vi "file -- accumulate data files -- V5.vi"(11 "list of <mmddyy> folders":path[](array[path])) -> (0 "timestamp (min) array":dbl[](array[numeric]), 2 "sweep file name  array":T1[](array[typedef]))   [LabVIEW 2015]
uses:
  sweep file name.ctl
  file -- scan filename action.ctl
  Split file name.vi
  find all matching strings in the list.vi
panel:
  in  "dummy":T1={"temperature"=0.0, "temperature str"="", "file path"=path "/snowfall/Users/arcadi/Desktop/Ultrasound/Experiment/YBCO_4/Round1/Sweep12/June_2011/062511/221.16400K_300_3100_001_062511.dat", "last mod"=timestamp(0 s since 1904-01-01), "file name str"="", "mod time(min)"=0.0, "file format"=enum."", "power(V)"=0.0, "Magn Field(T) "=0.0}
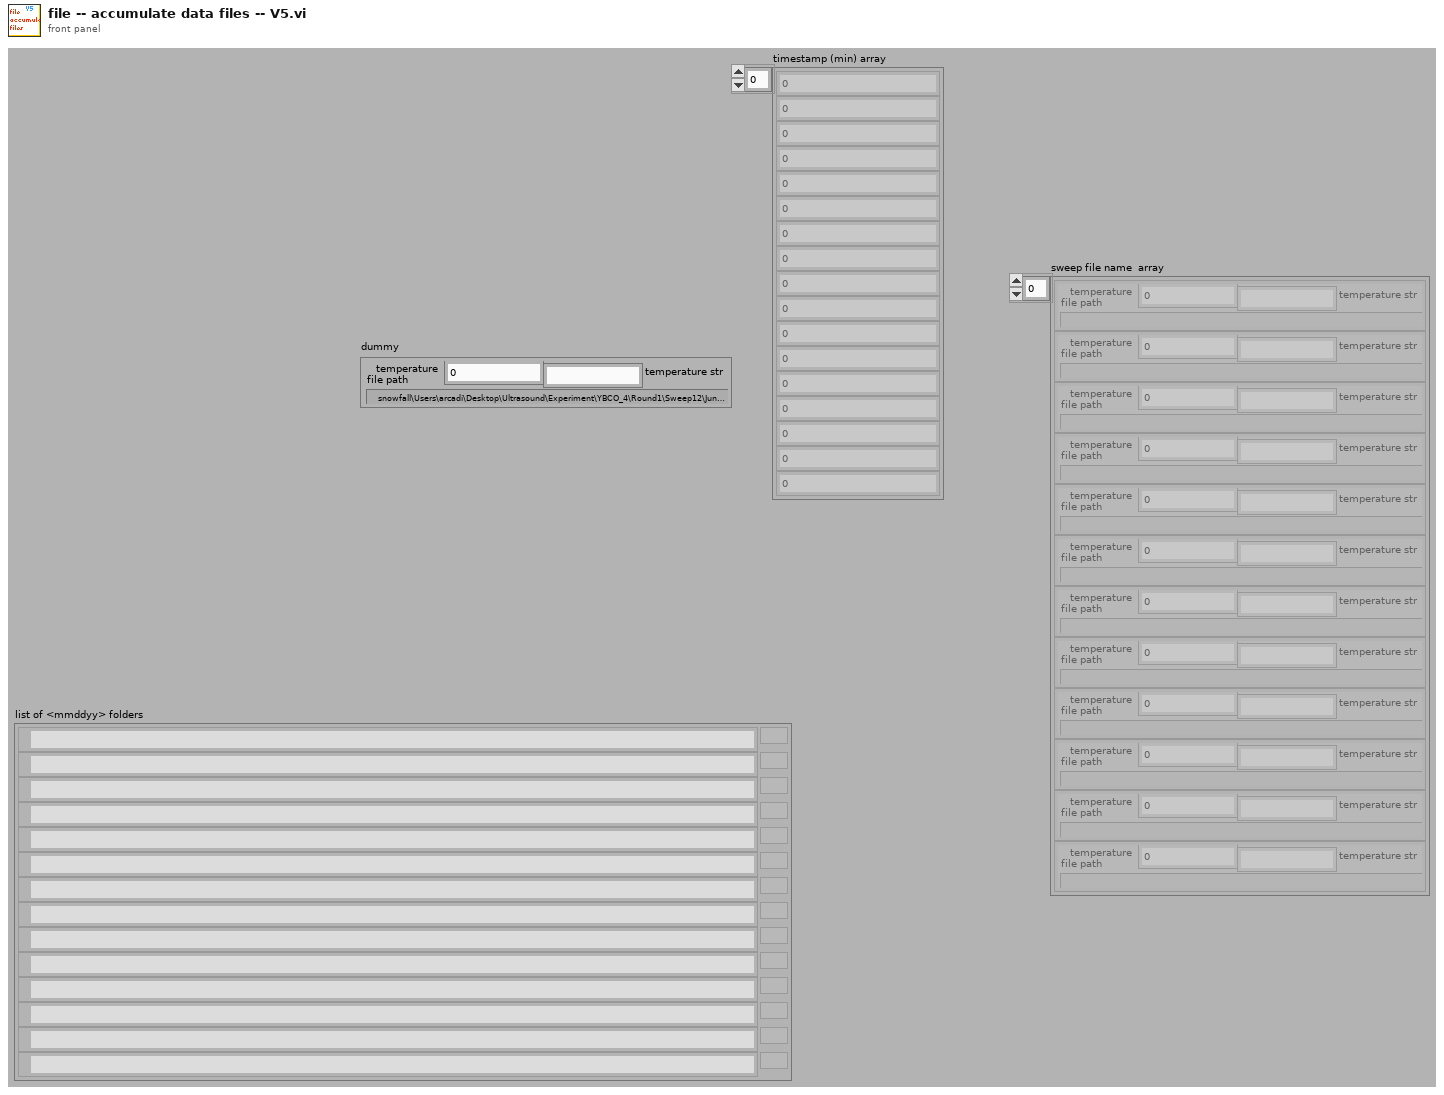
[diagram p1: front panel]
types:
  T1 = typedef "sweep file name.ctl" = cluster{"temperature":dbl, "temperature str":string, "file path":path, "last mod":timestamp, "file name str":string, "mod time(min)":dbl, "file format":enum16{"", "ascii", "binary"}, "power(V)":dbl, "Magn Field(T) ":dbl}
  T2 = typedef "file -- scan filename action.ctl" = enum16{"prefix base name", "datestring regexp", "parse datestring", "datestring", "filename regexp", "parse filename", "datestring regexp (no brackets)", "suffix base name"}
  T3 = cluster{"basename":string, "dat":bool, "bin":bool}[]
  T4 = typedef "file -- scan filename.ctl" = cluster{"mmddyy (str)":string, "counter (str)":string, "to F (kHz)":dbl, "from F (kHz)":dbl, "temperature (K)":dbl, "date/time string":string, "time stamp":timestamp, "base name":string, "temperature (str)":string, "from F (str)":string, "to F (str)":string, "format":enum16{"no date string", "with date string"}, "power (V)":dbl, "power (str) ":string, "Magn Field (T)":dbl, "Magn Field (str)":string}
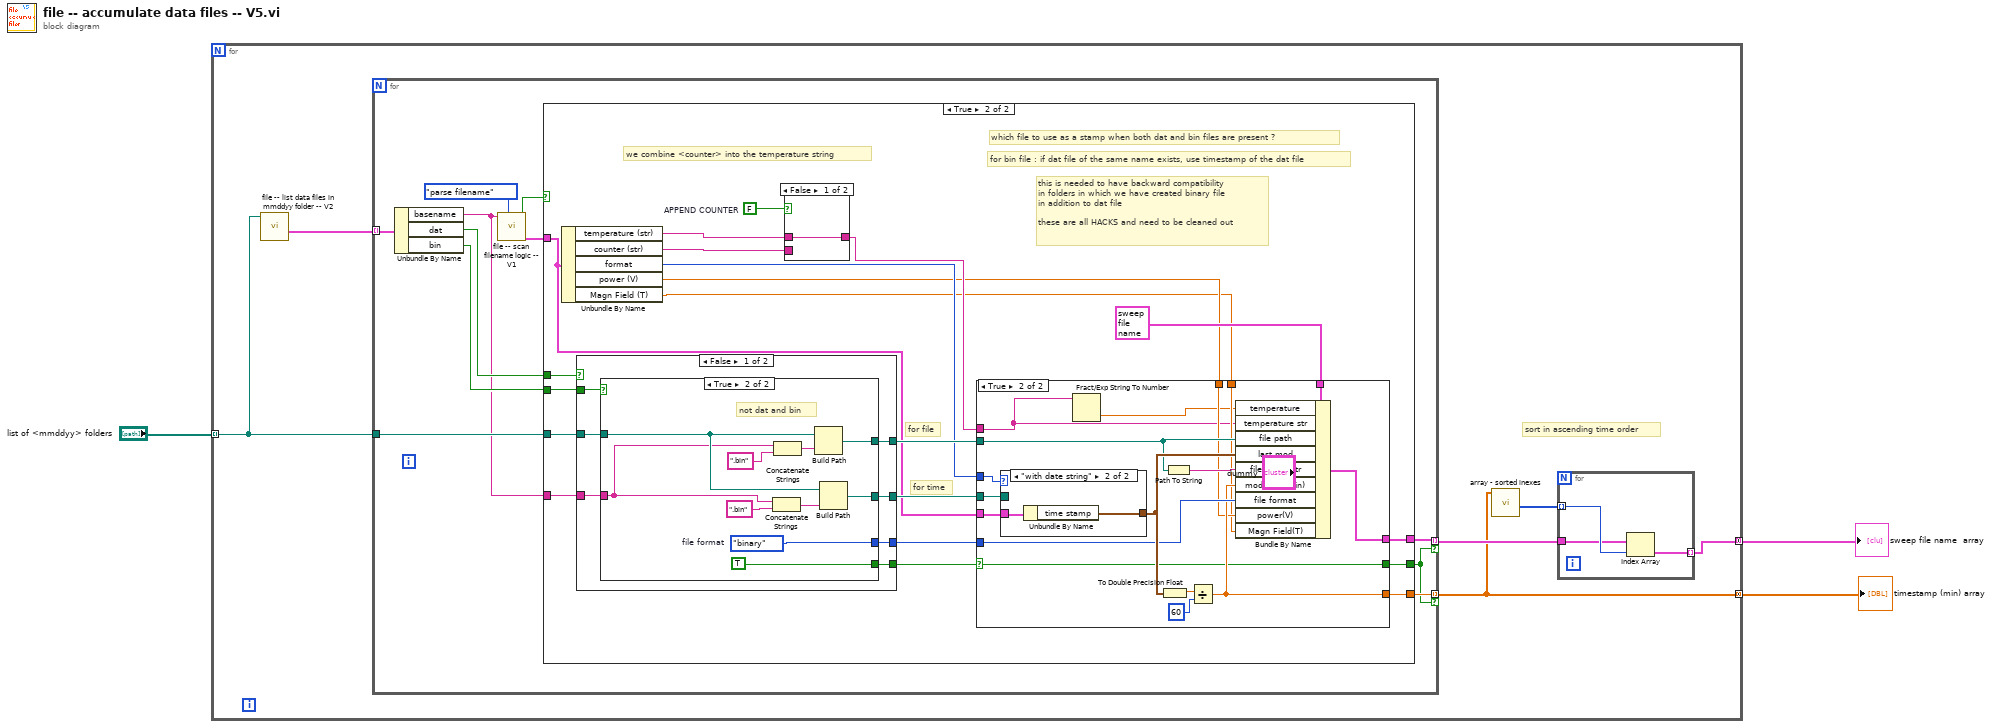
[diagram p0: block diagram]
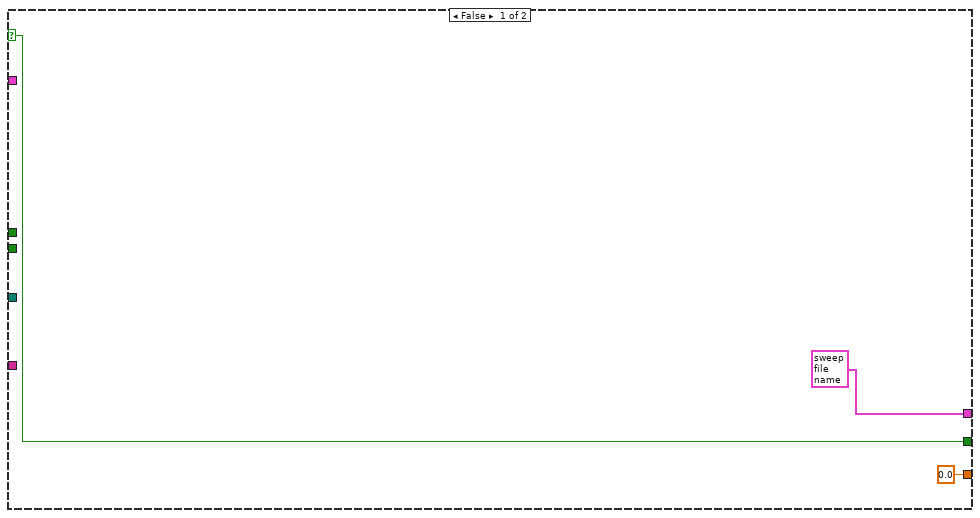
[diagram p2: hidden frame]
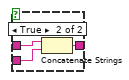
[diagram p3: hidden frame]
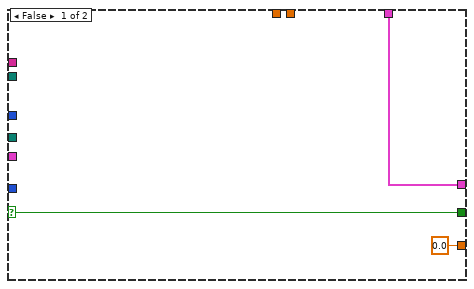
[diagram p4: hidden frame]
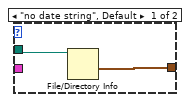
[diagram p5: hidden frame]
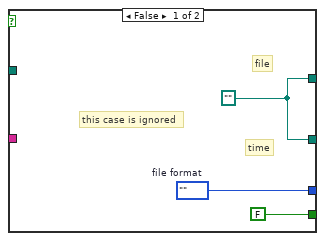
[diagram p6: hidden frame]
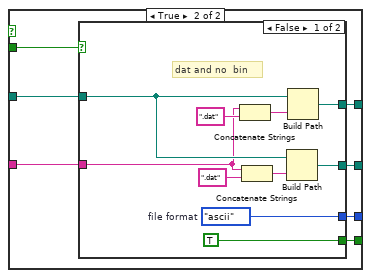
[diagram p7: hidden frame]
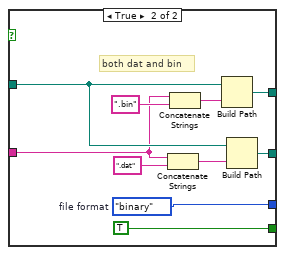
[diagram p8: hidden frame]
diagram:
  n1 = for {
    tunnel: "list of <mmddyy> folders" -> [w8] mode=indexing
    tunnel: [w5] -> w1 mode=concatenating
    tunnel: [w4] -> w2 mode=concatenating
    # "sort in ascending time order"
    n2 = call "file -- list data files in mmddyy folder -- V2.vi"("<mmddyy> folder path"=w8) -> ("Array"=w9:T3)  [unwired: 10 in]
    n3 = for {
      tunnel: w9 -> [w21] mode=indexing
      tunnel: w8 -> [w23]
      tunnel: [w14] -> w6 mode=indexing if=w13
      tunnel: [w22] -> w4 mode=indexing if=w13
      n4 = Unbundle By Name(w21) -> ("basename"=w17:string, "dat"=w19:bool, "bin"=w18:bool)
      n5 = call "file -- scan filename logic -- V1.vi"("scan fileneme action"=file_--_scan_filename_action."parse filename", "base name IN"=w17) -> ("scan filename OUT"=w16:T4, "exact match"=w20:bool)  [unwired: 7 in, 1 out]
      n6 = case shown="True" w20 {
        selector: w20 -> [w26 _]
        tunnel: w23 -> [_ w42]
        tunnel: [0.0 w46] -> w22
        tunnel: w16 -> [_ w33]
        tunnel: w19 -> [_ w44]
        tunnel: w18 -> [_ w43]
        tunnel: w17 -> [_ w41]
        tunnel: [T1 {"temperature"=0.0, "temperature str"="", "file path"=path "/snowfall/Users/arcadi/Desktop/Ultrasound/Experiment/YBCO_4/Round1/Sweep12/June_2011/062511/221.16400K_300_3100_001_062511.dat", "last mod"=timestamp(0 s since 1904-01-01), "file name str"="", "mod time(min)"=0.0, "file format"=enum."ascii", "power(V)"=0.0, "Magn Field(T) "=0.0} ("output cluster") w32] -> w14
        tunnel: [w26 w31] -> w13
        frame False {
        }
        frame True {
          w28 = FALSE  # APPEND COUNTER
          # "this is needed to have backward compatibility\nin folders in which we have created binary file\nin addition to dat file \n\nthese are all HACKS and need to be cleaned out"
          # "for file"
          # "for time"
          # "we combine <counter> into the temperature string"
          # "which file to use as a stamp when both dat and bin files are present ?"
          # "for bin file : if dat file of the same name exists, use timestamp of the dat file"
          n7 = Unbundle By Name(w33) -> ("temperature (str)"=w45:string, "counter (str)"=w35:string, "format"=w34:enum16{"no date string", "with date string"}, "power (V)"=w29:dbl, "Magn Field (T)"=w27:dbl)
          n8 = case shown="False" w44 {
            tunnel: w43 -> [w76 w101]
            tunnel: w42 -> [w78 w100]
            tunnel: w41 -> [w77 w99]
            tunnel: [w81 w98] -> w38
            tunnel: [w80 w97] -> w40
            tunnel: [w79 w96] -> w39
            tunnel: [w75 w95] -> w36
            frame False {
              n9 = case shown="True" w76 {
                tunnel: w78 -> [_ w90]
                tunnel: w77 -> [_ w89]
                tunnel: [w82 w93] -> w81
                tunnel: [w82 w88] -> w80
                tunnel: [w84 w86] -> w79
                tunnel: [FALSE ("quote specials") TRUE ("quote specials")] -> w75
                frame False {
                  w82 = path ""
                  w84 = enum16{"", "ascii", "binary"}.""  # file format
                  # "time"
                  # "file"
                  # "this case is ignored"
                }
                frame True {
                  w86 = enum16{"", "ascii", "binary"}."binary"  # file format
                  # "not dat and bin"
                  n10 = Concatenate Strings(w89, ".bin" ("string")) -> (w91:string)
                  n11 = Concatenate Strings(w89, ".bin" ("string")) -> (w87:string)
                  n12 = Build Path(base path=w90, name or relative path=w87) -> (appended path=w93:path)
                  n13 = Build Path(base path=w90, name or relative path=w91) -> (appended path=w88:path)
                }
              }
            }
            frame True {
              n14 = case shown="False" w101 {
                tunnel: w100 -> [w107 w117]
                tunnel: w99 -> [w103 w116]
                tunnel: [w106 w120] -> w98
                tunnel: [w105 w115] -> w97
                tunnel: [w104 w113] -> w96
                tunnel: [TRUE ("quote specials") TRUE ("quote specials")] -> w95
                frame False {
                  w104 = enum16{"", "ascii", "binary"}."ascii"  # file format
                  # "dat and no  bin"
                  n15 = Concatenate Strings(w103, ".dat" ("string")) -> (w108:string)
                  n16 = Concatenate Strings(w103, ".dat" ("string")) -> (w109:string)
                  n17 = Build Path(base path=w107, name or relative path=w109) -> (appended path=w105:path)
                  n18 = Build Path(base path=w107, name or relative path=w108) -> (appended path=w106:path)
                }
                frame True {
                  w113 = enum16{"", "ascii", "binary"}."binary"  # file format
                  # "both dat and bin"
                  n19 = Concatenate Strings(w116, ".dat" ("string")) -> (w118:string)
                  n20 = Concatenate Strings(w116, ".bin" ("string")) -> (w114:string)
                  n21 = Build Path(base path=w117, name or relative path=w114) -> (appended path=w120:path)
                  n22 = Build Path(base path=w117, name or relative path=w118) -> (appended path=w115:path)
                }
              }
            }
          }
          n23 = case shown="False" w28 {
            tunnel: w45 -> [w47 w50]
            tunnel: [w47 w49] -> w37
            tunnel: w35 -> [_ w48]
            frame False {
            }
            frame True {
              n24 = Concatenate Strings(w50, w48) -> (w49:string)
            }
          }
          n25 = case shown="True" w36 {
            selector: w36 -> [w53 w60]
            tunnel: [0.0 w61] -> w46
            tunnel: w40 -> [_ w67]
            tunnel: w39 -> [_ w66]
            tunnel: w38 -> [_ w65]
            tunnel: w37 -> [_ w55]
            tunnel: w34 -> [_ w63]
            tunnel: w33 -> [_ w62]
            tunnel: [w52 w59] -> w32
            tunnel: [w53 w60] -> w31
            tunnel: T1 {"temperature"=0.0, "temperature str"="", "file path"=path "/snowfall/Users/arcadi/Desktop/Ultrasound/Experiment/YBCO_4/Round1/Sweep12/June_2011/062511/221.16400K_300_3100_001_062511.dat", "last mod"=timestamp(0 s since 1904-01-01), "file name str"="", "mod time(min)"=0.0, "file format"=enum."ascii", "power(V)"=0.0, "Magn Field(T) "=0.0} ("output cluster") -> [w52 w58]
            tunnel: w29 -> [_ w57]
            tunnel: w27 -> [_ w56]
            frame False {
            }
            frame True {
              n26 = case shown="\"with date string\"" w63 {
                tunnel: [w72 w73] -> w70
                tunnel: w67 -> [w71 _]
                tunnel: w62 -> [_ w74]
                frame "no date string", Default {
                  n27 = File/Directory Info(path=w71) -> (last mod=w72:timestamp)  [unwired: 1 in, 6 out]
                }
                frame "with date string" {
                  n28 = Unbundle By Name(w74) -> ("time stamp"=w73:timestamp)
                }
              }
              n29 = Fract/Exp String To Number(string=w55) -> (number=w54:dbl)  [unwired: 3 in, 1 out]
              n30 = To Double Precision Float(number=w70) -> (double precision float=w69:dbl)
              n31 = Path To String(path=w65) -> (string=w64:string)
              n32 = Divide(x=w69, y=60) -> (x/y=w61:dbl)
              n33 = Bundle By Name(cluster=w58, "temperature"=w54, "temperature str"=w55, "file path"=w65, "last mod"=w70, "file name str"=w64, "mod time(min)"=w61, "file format"=w66, "power(V)"=w57, "Magn Field(T)"=w56) -> (w59:T1)
            }
          }
        }
      }
    }
    n34 = call "array - sorted inexes.vi"("x"=w4) -> ("index array"=w7:i32[])  [unwired: 9 in, 1 out]
    n35 = for {
      tunnel: w7 -> [w11] mode=indexing
      tunnel: [w12] -> w5 mode=indexing
      tunnel: w6 -> [w10]
      n36 = Index Array(array=w10, index=w11) -> (element=w12:T1)
    }
  }
  "sweep file name  array" <- w1
  "timestamp (min) array" <- w2
